vi "Modbus FVIR Sensors.vi"(8 "error in":errorcluster, 11 "PLC Data":T1) -> (0 "error out":errorcluster, 3 "PLC Data Out":T1)   [LabVIEW 2020, in "Modbus.lvlib"]
uses:
  Modbus.lvlib
  Modbus PLC Data All.ctl
  Modbus FVIR Control.ctl
  Modbus LDO Control.ctl
  WritingDataFile/Data to Save.ctl
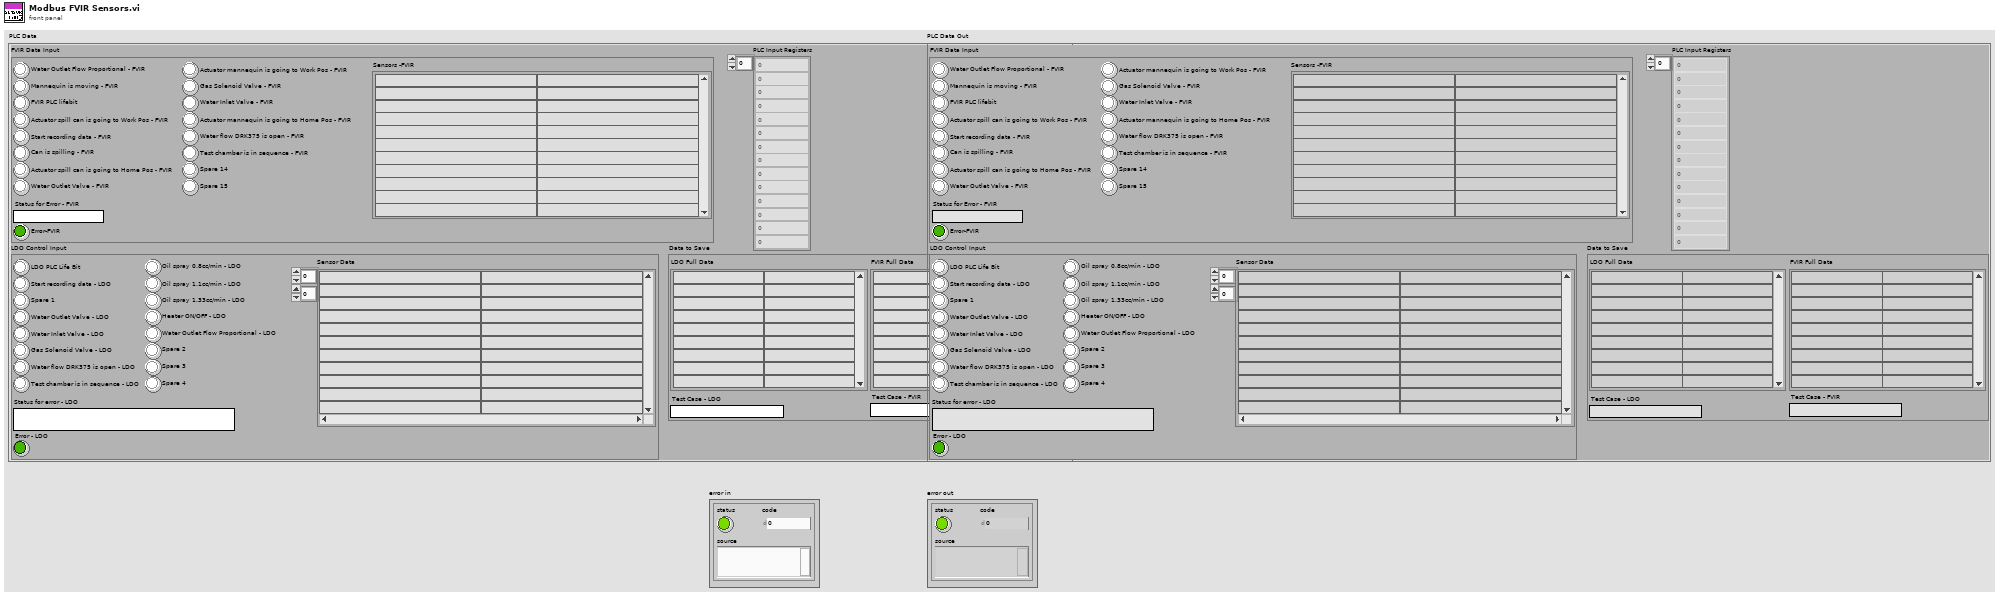
[diagram p1: front panel]
types:
  T1 = typedef "Modbus PLC Data All.ctl" = cluster{"FVIR Data Input":T2, "LDO Control Input":T3, "PLC Input Registers":u16[], "Data to Save":T4}
  T2 = typedef "Modbus FVIR Control.ctl" = cluster{"Spare 15":bool, "Spare 14":bool, "Actuator mannequin is going to Work Pos - FVIR":bool, "Actuator mannequin is going to Home Pos - FVIR":bool, "Test chamber is in sequence - FVIR ":bool, "Water flow DRK375 is open - FVIR":bool, "Gas Solenoid Valve - FVIR":bool, "Water Inlet Valve - FVIR":bool, "Water Outlet Flow Proportional - FVIR":bool, "Start recording data - FVIR":bool, "Actuator spill can is going to Work Pos - FVIR":bool, "Actuator spill can is going to Home Pos - FVIR":bool, "Water Outlet Valve - FVIR":bool, "Can is spilling - FVIR":bool, "Mannequin is moving - FVIR":bool, "FVIR PLC lifebit":bool, "Status for Error - FVIR":string, "Error-FVIR":bool, "Sensors -FVIR":string[][]}
  T3 = typedef "Modbus LDO Control.ctl" = cluster{"LDO PLC Life Bit":bool, "Start recording data - LDO":bool, "Spare 1":bool, "Water Outlet Valve - LDO":bool, "Water Inlet Valve - LDO":bool, "Gas Solenoid Valve - LDO":bool, "Water flow DRK375 is open - LDO":bool, "Test chamber is in sequence - LDO":bool, "Oil spray 0.8cc/min - LDO":bool, "Oil spray 1.1cc/min - LDO":bool, "Oil spray 1.33cc/min - LDO":bool, "Heater ON/OFF - LDO":bool, "Water Outlet Flow Proportional - LDO":bool, "Spare 2":bool, "Spare 3":bool, "Spare 4":bool, "Status for error - LDO":string, "Error - LDO":bool, "Sensor Data":string[][]}
  T4 = typedef "Data to Save.ctl" = cluster{"LDO Full Data":string[][], "FVIR Full Data":string[][], "Test Case - FVIR":string, "Test Case - LDO":string}
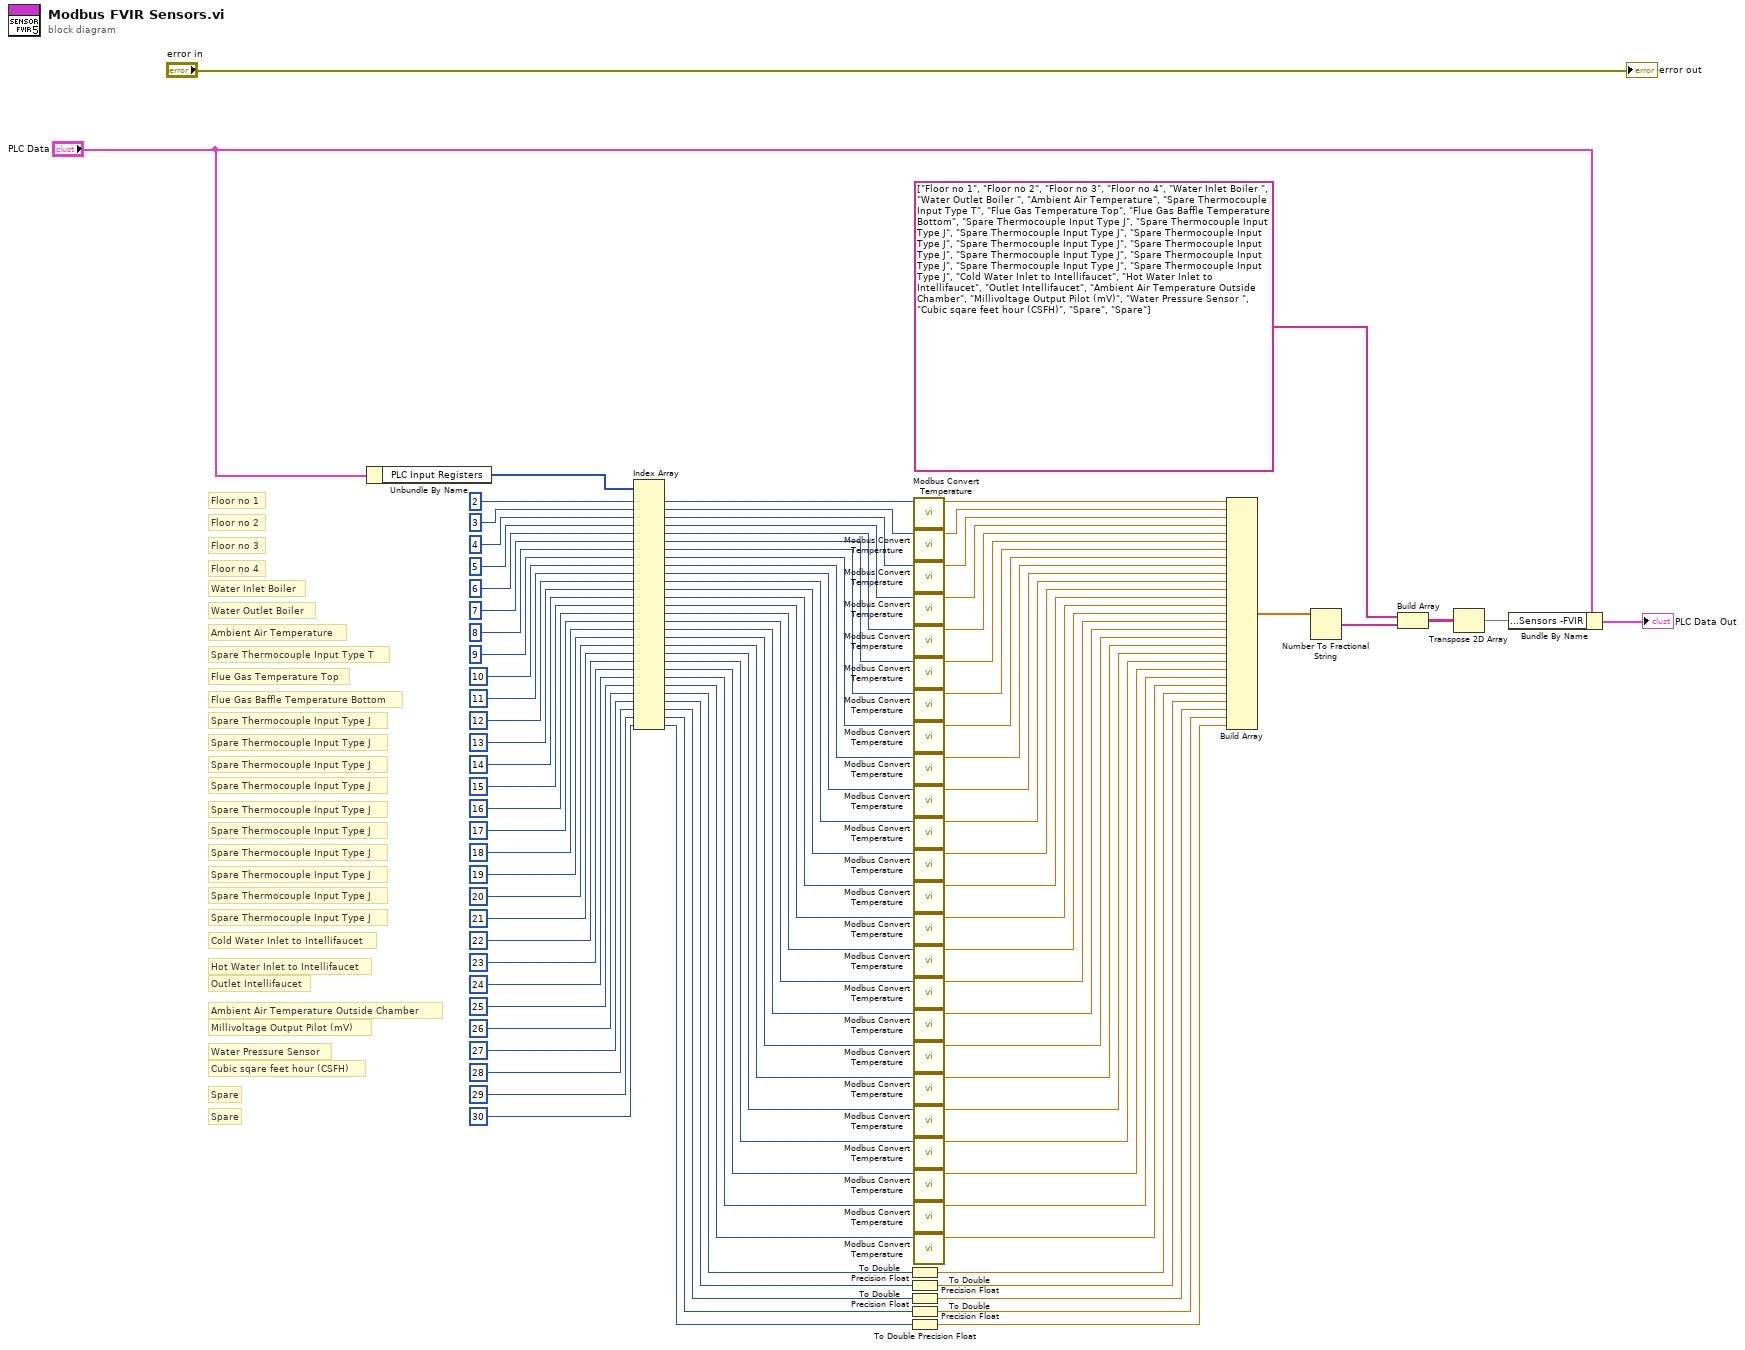
[diagram p0: block diagram]
diagram:
  # "Spare"
  # "Spare"
  # "Cubic sqare feet hour (CSFH)"
  # "Water Pressure Sensor"
  # "Millivoltage Output Pilot (mV)"
  # "Ambient Air Temperature Outside Chamber"
  # "Outlet Intellifaucet"
  # "Hot Water Inlet to Intellifaucet"
  # "Cold Water Inlet to Intellifaucet"
  # "Spare Thermocouple Input Type J"
  # "Spare Thermocouple Input Type J"
  # "Spare Thermocouple Input Type J"
  # "Spare Thermocouple Input Type J"
  # "Spare Thermocouple Input Type J"
  # "Spare Thermocouple Input Type J"
  # "Spare Thermocouple Input Type J"
  # "Spare Thermocouple Input Type J"
  # "Spare Thermocouple Input Type J"
  # "Spare Thermocouple Input Type J"
  # "Flue Gas Baffle Temperature Bottom"
  # "Flue Gas Temperature Top"
  # "Spare Thermocouple Input Type T"
  # "Ambient Air Temperature"
  # "Water Outlet Boiler"
  # "Water Inlet Boiler"
  # "Floor no 4"
  # "Floor no 3"
  # "Floor no 2"
  # "Floor no 1"
  n1 = Unbundle By Name("PLC Data") -> ("PLC Input Registers"=w3:u16[])
  n2 = Index Array(array=w3, index #1=2 ("index"), index #2=3 ("index"), index #3=4 ("index"), index #4=5 ("index"), index #5=6 ("index"), index #6=7 ("index"), index #7=8 ("index"), index #8=9 ("index"), index #9=10 ("index"), index #10=11 ("index"), index #11=12 ("index"), index #12=13 ("index"), index #13=14 ("index"), index #14=15 ("index"), index #15=16 ("index"), index #16=17 ("index"), index #17=18 ("index"), index #18=19 ("index"), index #19=20 ("index"), index #20=21 ("index"), index #21=22 ("index"), index #22=23 ("index"), index #23=24 ("index"), index #24=25 ("index"), index #25=26 ("index"), index #26=27 ("index"), index #27=28 ("index"), index #28=29 ("index"), index #29=30 ("index")) -> (element #1=w66:u16, element #2=w65:u16, element #3=w64:u16, element #4=w63:u16, element #5=w62:u16, element #6=w61:u16, element #7=w60:u16, element #8=w59:u16, element #9=w58:u16, element #10=w57:u16, element #11=w56:u16, element #12=w55:u16, element #13=w54:u16, element #14=w53:u16, element #15=w52:u16, element #16=w51:u16, element #17=w50:u16, element #18=w49:u16, element #19=w48:u16, element #20=w47:u16, element #21=w46:u16, element #22=w45:u16, element #23=w44:u16, element #24=w43:u16, element #25=w10:u16, element #26=w12:u16, element #27=w14:u16, element #28=w16:u16, element #29=w18:u16)
  n3 = To Double Precision Float(number=w10) -> (double precision float=w9:dbl)
  n4 = To Double Precision Float(number=w12) -> (double precision float=w11:dbl)
  n5 = To Double Precision Float(number=w14) -> (double precision float=w13:dbl)
  n6 = To Double Precision Float(number=w16) -> (double precision float=w15:dbl)
  n7 = To Double Precision Float(number=w18) -> (double precision float=w17:dbl)
  n8 = call "Modbus Convert Temperature.vi"("PLC Value"=w66) -> ("Converted Value"=w42:dbl)  [unwired: 9 in, 1 out]
  n9 = call "Modbus Convert Temperature.vi"("PLC Value"=w65) -> ("Converted Value"=w41:dbl)  [unwired: 9 in, 1 out]
  n10 = call "Modbus Convert Temperature.vi"("PLC Value"=w64) -> ("Converted Value"=w40:dbl)  [unwired: 9 in, 1 out]
  n11 = call "Modbus Convert Temperature.vi"("PLC Value"=w63) -> ("Converted Value"=w39:dbl)  [unwired: 9 in, 1 out]
  n12 = call "Modbus Convert Temperature.vi"("PLC Value"=w62) -> ("Converted Value"=w38:dbl)  [unwired: 9 in, 1 out]
  n13 = call "Modbus Convert Temperature.vi"("PLC Value"=w61) -> ("Converted Value"=w37:dbl)  [unwired: 9 in, 1 out]
  n14 = call "Modbus Convert Temperature.vi"("PLC Value"=w60) -> ("Converted Value"=w36:dbl)  [unwired: 9 in, 1 out]
  n15 = call "Modbus Convert Temperature.vi"("PLC Value"=w59) -> ("Converted Value"=w35:dbl)  [unwired: 9 in, 1 out]
  n16 = call "Modbus Convert Temperature.vi"("PLC Value"=w58) -> ("Converted Value"=w34:dbl)  [unwired: 9 in, 1 out]
  n17 = call "Modbus Convert Temperature.vi"("PLC Value"=w57) -> ("Converted Value"=w33:dbl)  [unwired: 9 in, 1 out]
  n18 = call "Modbus Convert Temperature.vi"("PLC Value"=w56) -> ("Converted Value"=w32:dbl)  [unwired: 9 in, 1 out]
  n19 = call "Modbus Convert Temperature.vi"("PLC Value"=w55) -> ("Converted Value"=w31:dbl)  [unwired: 9 in, 1 out]
  n20 = call "Modbus Convert Temperature.vi"("PLC Value"=w54) -> ("Converted Value"=w30:dbl)  [unwired: 9 in, 1 out]
  n21 = call "Modbus Convert Temperature.vi"("PLC Value"=w53) -> ("Converted Value"=w29:dbl)  [unwired: 9 in, 1 out]
  n22 = call "Modbus Convert Temperature.vi"("PLC Value"=w52) -> ("Converted Value"=w28:dbl)  [unwired: 9 in, 1 out]
  n23 = call "Modbus Convert Temperature.vi"("PLC Value"=w51) -> ("Converted Value"=w27:dbl)  [unwired: 9 in, 1 out]
  n24 = call "Modbus Convert Temperature.vi"("PLC Value"=w50) -> ("Converted Value"=w26:dbl)  [unwired: 9 in, 1 out]
  n25 = call "Modbus Convert Temperature.vi"("PLC Value"=w49) -> ("Converted Value"=w25:dbl)  [unwired: 9 in, 1 out]
  n26 = call "Modbus Convert Temperature.vi"("PLC Value"=w48) -> ("Converted Value"=w24:dbl)  [unwired: 9 in, 1 out]
  n27 = call "Modbus Convert Temperature.vi"("PLC Value"=w47) -> ("Converted Value"=w23:dbl)  [unwired: 9 in, 1 out]
  n28 = call "Modbus Convert Temperature.vi"("PLC Value"=w46) -> ("Converted Value"=w22:dbl)  [unwired: 9 in, 1 out]
  n29 = call "Modbus Convert Temperature.vi"("PLC Value"=w45) -> ("Converted Value"=w21:dbl)  [unwired: 9 in, 1 out]
  n30 = call "Modbus Convert Temperature.vi"("PLC Value"=w44) -> ("Converted Value"=w20:dbl)  [unwired: 9 in, 1 out]
  n31 = call "Modbus Convert Temperature.vi"("PLC Value"=w43) -> ("Converted Value"=w19:dbl)  [unwired: 9 in, 1 out]
  n32 = Build Array(w42, w41, w40, w39, w38, w37, w36, w35, w34, w33, w32, w31, w30, w29, w28, w27, w26, w25, w24, w23, w22, w21, w20, w19, w9, w11, w13, w15, w17) -> (w6:dbl[])
  n33 = Number To Fractional String(number=w6) -> (F-format string=w7:string[])  [unwired: 3 in]
  n34 = Build Array(string[] ["Floor no 1", "Floor no 2", "Floor no 3", "Floor no 4", "Water Inlet Boiler ", "Water Outlet Boiler ", "Ambient Air Temperature", "Spare Thermocouple Input Type T", "Flue Gas Temperature Top", "Flue Gas Baffle Temperature Bottom", "Spare Thermocouple Input Type J", "Spare Thermocouple Input Type J", "Spare Thermocouple Input Type J", "Spare Thermocouple Input Type J", "Spare Thermocouple Input Type J", "Spare Thermocouple Input Type J", "Spare Thermocouple Input Type J", "Spare Thermocouple Input Type J", "Spare Thermocouple Input Type J", "Spare Thermocouple Input Type J", "Cold Water Inlet to Intellifaucet", "Hot Water Inlet to Intellifaucet", "Outlet Intellifaucet", "Ambient Air Temperature Outside Chamber", "Millivoltage Output Pilot (mV)", "Water Pressure Sensor ", "Cubic sqare feet hour (CSFH)", "Spare", "Spare"], w7) -> (w8:string[][])
  n35 = Transpose 2D Array(2D array=w8) -> (transposed array=w4:string[][])
  n36 = Bundle By Name(cluster="PLC Data", "FVIR Data Input.Sensors -FVIR"=w4) -> (→"PLC Data Out":T1)
  "error out" <- "error in"
